vi "Configure Overvoltage Protection.vi"(0 "VISA resource name":refnum<visa-resource-name>, 5 "Enable Overvoltage Protection (F: Disable)":bool, 7 "Overvoltage Protection Threshold (500 V)":dbl=500.0 format="%#.4g", 9 "Overvoltage Protection Delay (0.1 s)":dbl=0.1 format="%^#.4g", 11 "error in (no error)":errorcluster) -> (4 "VISA resource name out":refnum<visa-resource-name>, 15 "error out":errorcluster)   [LabVIEW 2020, in "Agilent 681x Series.lvlib"]
doc: "Configures the overvoltage protection settings of the instrument."
uses:
  <instrlib>/Agilent 681x Series/Agilent 681x Series.lvlib
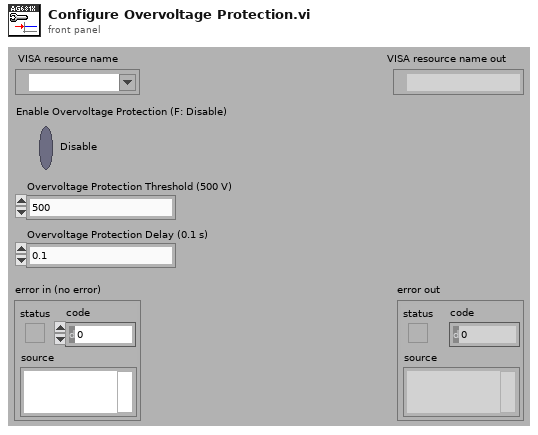
[diagram p1: front panel]
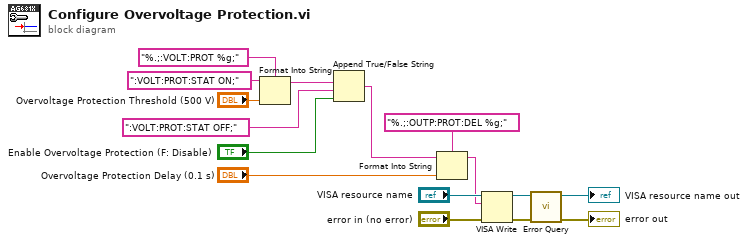
[diagram p0: block diagram]
diagram:
  n1 = Format Into String(format string="%.;:VOLT:PROT %g;", initial string=":VOLT:PROT:STAT ON;", "Overvoltage Protection Threshold (500 V)") -> (resulting string=w6:string)  [unwired: 1 in, 1 out]
  n2 = Append True/False String(1:"Enable Overvoltage Protection (F: Disable)", 2:":VOLT:PROT:STAT OFF;" ("false string"), 3:w6) -> (0:w1:string)  [unwired: 1 in]
  n3 = Format Into String(format string="%.;:OUTP:PROT:DEL %g;", initial string=w1, "Overvoltage Protection Delay (0.1 s)") -> (resulting string=w3:string)  [unwired: 1 in, 1 out]
  n4 = VISA Write(VISA resource name="VISA resource name", write buffer=w3, error in (no error)="error in (no error)") -> (VISA resource name out=w14:refnum<visa-resource-name>, error out=w13:errorcluster)  [unwired: 1 out]
  n5 = call <instrlib>:"Error Query.vi"("error in (no error)"=w13, "VISA resource name"=w14) -> ("error out"=→"error out":errorcluster, "VISA resource name out"=→"VISA resource name out":refnum<visa-resource-name>)  [unwired: 6 in, 2 out]
